vi "GetCustomDeviceXMLVIs.vi"(8 "error in (no error)":errorcluster, 11 "absolute custom device xml file":path) -> (0 "error out":errorcluster, 3 "custom device VIs":T1(array[cluster]))   [LabVIEW 2016, in "VeriStandTestUtilities.lvlib"]
uses:
  VeriStandTestUtilities.lvlib
  NationalInstruments.VeriStand.SystemStorage
  NationalInstruments.VeriStand.XMLReader
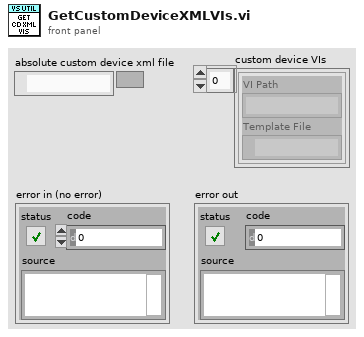
[diagram p1: front panel]
types:
  T1 = cluster{"VI Path":string, "Template File":path}[]
  T2 = cluster{"Item2Launch":refnum<k24>, "Template File":path}
  T3 = cluster{"Item2Launch":refnum<k24>, "Template File":path}[]
  T4 = cluster{"Source":refnum<k24>, "Folder Path":path}[]
  T5 = cluster{"Location":refnum<k24>, "Folder Path":path}[]
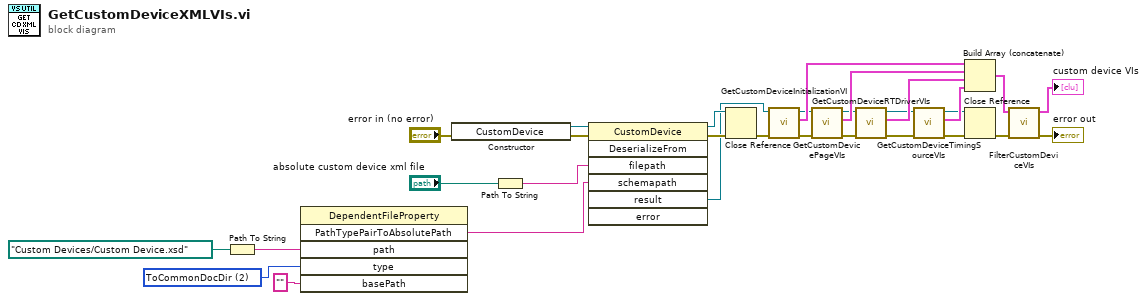
[diagram p0: block diagram]
diagram:
  w22 = 2 items=["Absolute", "Relative", "ToCommonDocDir", "ToApplicationDataDir"] ("type")
  n1 = Path To String(path=path "Custom Devices/Custom Device.xsd") -> (string=w24:string)
  n2 = invoke class="DependentFileProperty" method="PathTypePairToAbsolutePath"("path"=w24, "type"=w22, "basePath"="") -> ("PathTypePairToAbsolutePath"=w19:string)  [unwired: 3 in, 5 out]
  n3 = constructor class="CustomDevice"(error in="error in (no error)") -> (reference out=w28:refnum<k24>, error out=w29:errorcluster)  [unwired: 2 in, 1 out]
  n4 = Path To String(path="absolute custom device xml file") -> (string=w26:string)
  n5 = invoke class="CustomDevice" method="DeserializeFrom"(reference=w28, error in=w29, "filepath"=w26, "schemapath"=w19) -> (reference out=w20:refnum<k24>, error out=w21:errorcluster, "result"=w7:refnum<k24>)  [unwired: 3 in, 4 out]
  n6 = Close Reference(reference=w20, error in (no error)=w21) -> (error out=w5:errorcluster)
  n7 = call "GetCustomDeviceInitializationVI.vi"("error in (no error)"=w5, "custom device reference in"=w7) -> ("error out"=w11:errorcluster, "initialization VI"=w16:T2, "custom device reference out"=w10:refnum<k24>)  [unwired: 7 in]
  n8 = call "GetCustomDevicePageVIs.vi"("error in (no error)"=w11, "custom device reference in"=w10) -> ("error out"=w12:errorcluster, "page VIs"=w15:T3, "custom device reference out"=w9:refnum<k24>)  [unwired: 7 in]
  n9 = call "GetCustomDeviceRTDriverVIs.vi"("error in (no error)"=w12, "custom device reference in"=w9) -> ("error out"=w4:errorcluster, "RT driver VIs"=w14:T4, "custom device reference out"=w2:refnum<k24>)  [unwired: 7 in]
  n10 = call "GetCustomDeviceTimingSourceVIs.vi"("error in (no error)"=w4, "custom device reference in"=w2) -> ("error out"=w3:errorcluster, "timing source VIs"=w6:cluster{"Location":refnum<k24>, path}[], "custom device reference out"=w1:refnum<k24>)  [unwired: 7 in]
  n11 = Build Array (concatenate)(w16, w15, w14, w6) -> (w13:T5)
  n12 = Close Reference(reference=w1, error in (no error)=w3) -> (error out=w8:errorcluster)
  n13 = call "FilterCustomDeviceVIs.vi"("error in (no error)"=w8, "custom device VIs in"=w13) -> ("error out"=→"error out":errorcluster, "custom device VIs out"=→"custom device VIs":cluster{"Path1":string, "appended path":path}[])  [unwired: 8 in]
